vi "Get Is Door Open.vi"(8 "error in (no error)":errorcluster, 11 "Timed Door in":refnum<class "Timed Door.lvclass">) -> (0 "error out":errorcluster, 2 "Is Door Open?":bool, 3 "Timed Door out":refnum<class "Timed Door.lvclass">)   [LabVIEW 2018, in "Timed Door.lvclass"]
uses:
  Timed Door.lvclass
  Timed Door.lvclass/Timed Door.ctl
  Door/Door.lvclass
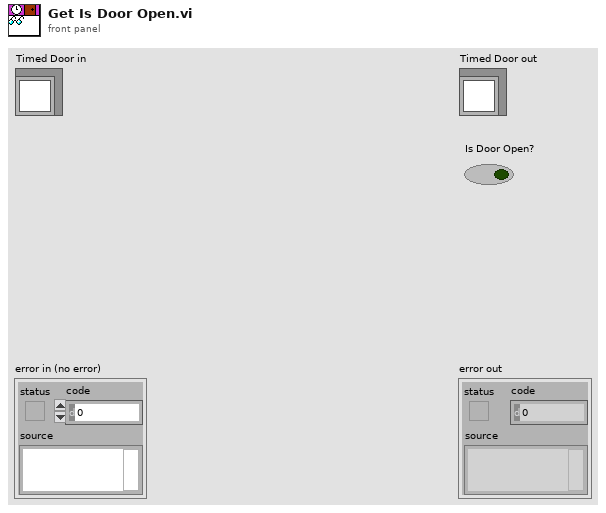
[diagram p1: front panel]
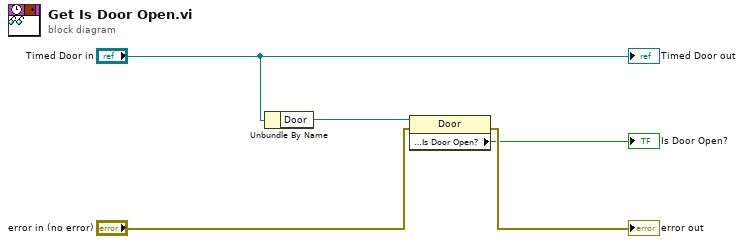
[diagram p0: block diagram]
diagram:
  n1 = Unbundle By Name("Timed Door in") -> ("Door"=w3:refnum<class "Door.lvclass">)
  n2 = property class="Door"(reference=w3, error in="error in (no error)") -> (error out=→"error out":errorcluster, "Accessors:Is Door Open?"=→"Is Door Open?":bool)  [unwired: 1 out]
  "Timed Door out" <- "Timed Door in"
